vi "UI IO Page.vi"(8 "error in":errorcluster) -> (0 "error out":errorcluster)   [LabVIEW 2019, in "UIs.lvlib"]
uses:
  UIs.lvlib
  <vilib>/Utility/miscctls.llb/LVPointTypeDef.ctl
  LED/SubVI/ADC Channel.ctl
  Controller/Controller.lvlib
  IO/sbRIO9623/sbRIO9623.lvlib
  Selection Valve/IDEX/IDEX.lvlib
  Syringe Pump/NE-500/NE-500.lvlib
  LED/LED.lvlib
panel:
  out "Syringe Pump Status":string
  out "Force Sensor 2":u32
  out "Force Sensor 1":u32
  out "Air Pressure (V)":dbl format="%#_2g"
  out "Blood Sensor 2 (V)":dbl format="%#_2g"
  out "Blood Sensor 1 (V)":dbl format="%#_2g"
  out "BL1 (V)":dbl format="%#_2g"
  out "BL2 (V)":dbl format="%#_2g"
  in  "Back":bool
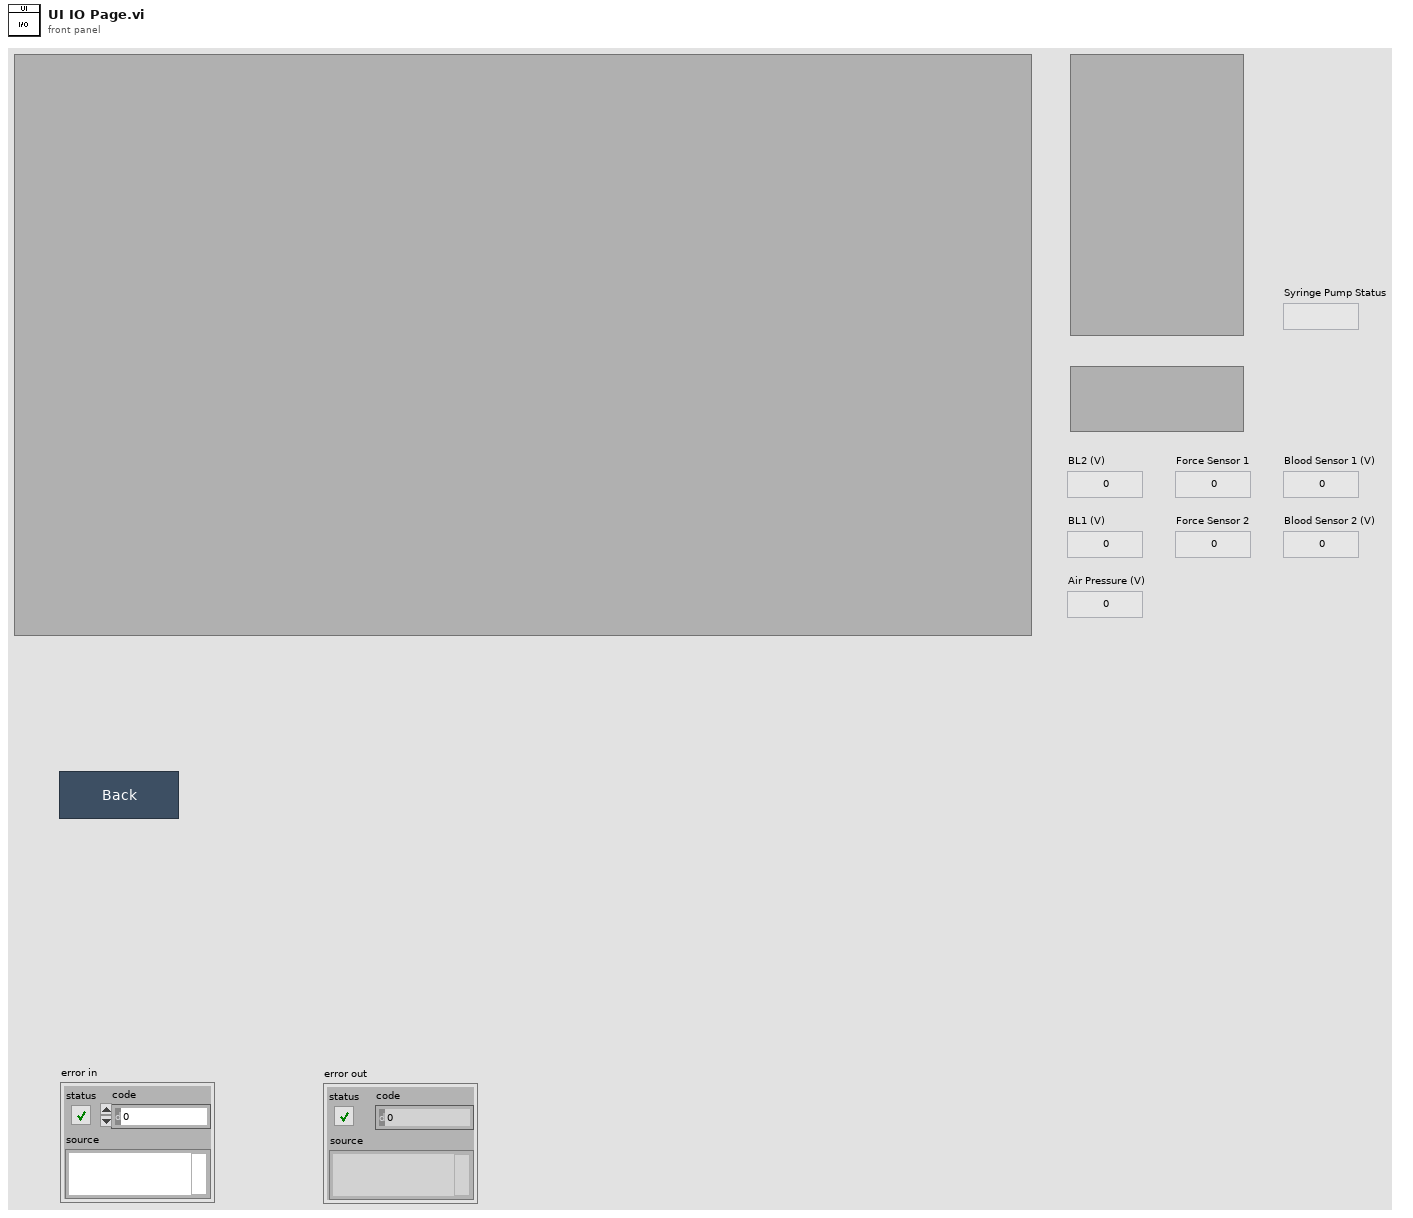
[diagram p1: front panel]
types:
  T1 = typedef "LVPointTypeDef.ctl" = cluster{"Horizontal":i16, "Vertical":i16}
  T2 = typedef "NE-500.lvlib/SEQ Data.ctl" = cluster{"Status":string, "Initialize Done?":bool, "VI Refnum":refnum<vi>}
  T3 = typedef "sbRIO9623.lvlib/SEQ Data.ctl" = cluster{"Lid Sensor 1":bool, "Lid Sensor 2":bool, "Laser Interlock":bool, "Buffer Tank":bool, "Wash Tank":bool, "Waste Tank":bool, "SiPM 1":fxp<+,20,5>, "SiPM 2":fxp<+,20,5>, "Initialize Success?":bool, "VI Refnum":refnum<vi>}
  T4 = typedef "IDEX.lvlib/SEQ Data.ctl" = cluster{"Position":string, "Initialize Done?":bool, "VI Refnum":refnum<vi>}
  T5 = typedef "LED.lvlib/ADC Channel.ctl" = enum16{"BL2 Regulator", "BL1 Regulator", "Blood Sensor 1", "Blood Sensor 2", "Air Pressure Sensor", "Force Sensor 1", "Force Snesor 2"}
  T6 = typedef "LED.lvlib/SEQ Data.ctl" = cluster{"Initialize Sucess?":bool, "BL2 Regulator":dbl, "BL1 Regulator":dbl, "Blood Sensor 1":dbl, "Blood Sensor 2":dbl, "Air Pressure Sensor":dbl, "Force Snesor 1":u32, "Force Snesor 2":u32, "VI Refnum":refnum<vi>}
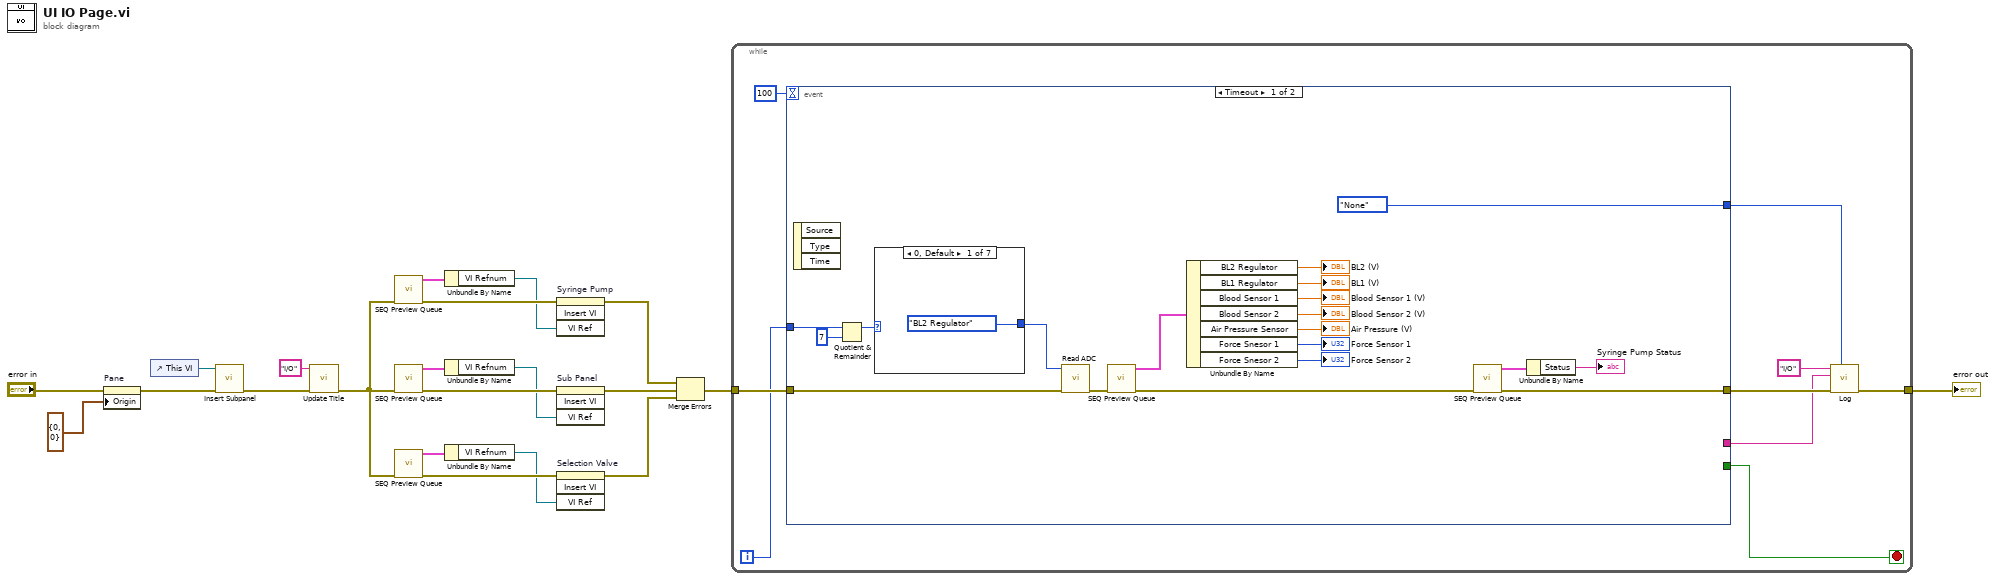
[diagram p0: block diagram]
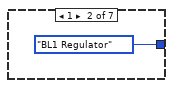
[diagram p2: hidden frame]
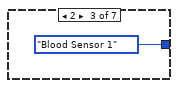
[diagram p3: hidden frame]
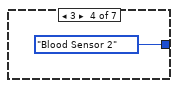
[diagram p4: hidden frame]
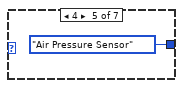
[diagram p5: hidden frame]
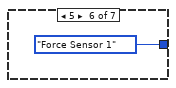
[diagram p6: hidden frame]
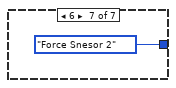
[diagram p7: hidden frame]
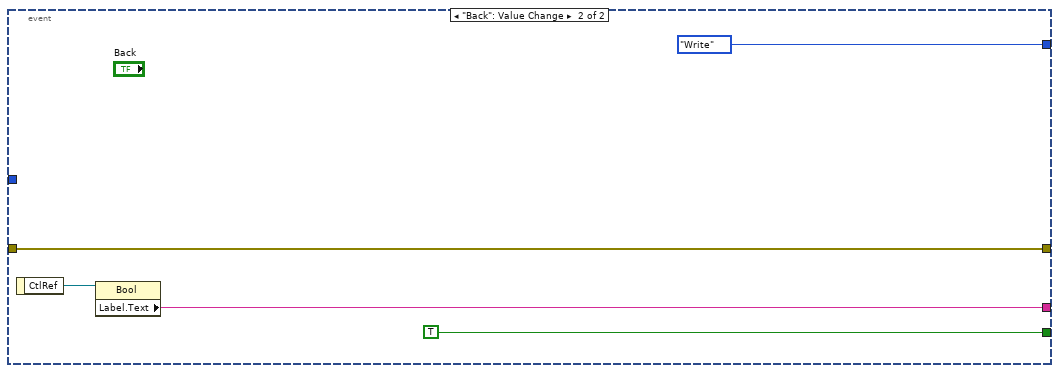
[diagram p8: hidden frame]
diagram:
  n1 = property on="Pane" class="Pane"(error in="error in", "Origin"=T1 {"Horizontal"=0, "Vertical"=0}) -> (error out=w15:errorcluster)  [unwired: 1 in, 1 out]
  n2 = control-ref of="This VI"() -> (w21:refnum<vi>)
  n3 = call "Insert Subpanel.vi"("Error In"=w15, "VI Refnum"=w21) -> ("Error Out"=w13:errorcluster)  [unwired: 9 in]
  n4 = call "Update Title.vi"("Error In"=w13, "Title"="I/O") -> ("Error Out"=w10:errorcluster)  [unwired: 9 in]
  n5 = call "SEQ Preview Queue.vi"("error in"=w10) -> ("error out"=w11:errorcluster, "SEQ Data"=w9:T2)  [unwired: 9 in]
  n6 = call "SEQ Preview Queue.vi"("error in"=w10) -> ("error out"=w19:errorcluster, "SEQ Data"=w20:T3)  [unwired: 9 in]
  n7 = call "SEQ Preview Queue.vi"("error in"=w10) -> ("error out"=w7:errorcluster, "SEQ Data"=w6:T4)  [unwired: 9 in]
  n8 = Unbundle By Name(w9) -> ("VI Refnum"=w8:refnum<vi>)
  n9 = Unbundle By Name(w20) -> ("VI Refnum"=w18:refnum<vi>)
  n10 = Unbundle By Name(w6) -> ("VI Refnum"=w5:refnum<vi>)
  n11 = invoke on="Syringe Pump" class="SubPnl" method="Insert VI"(error in=w11, "VI Ref"=w8) -> (error out=w4:errorcluster)  [unwired: 2 in, 3 out]
  n12 = invoke on="Sub Panel" class="SubPnl" method="Insert VI"(error in=w19, "VI Ref"=w18) -> (error out=w3:errorcluster)  [unwired: 2 in, 3 out]
  n13 = invoke on="Selection Valve" class="SubPnl" method="Insert VI"(error in=w7, "VI Ref"=w5) -> (error out=w2:errorcluster)  [unwired: 2 in, 3 out]
  n14 = Merge Errors(w4, w3, w2) -> (w1:errorcluster)
  n15 = while {
    tunnel: w1 -> [w30]
    tunnel: [w25] -> w17
    i -> [w28]
    stop <- w29 stop-if-true
    n16 = event shown="[0] Timeout" {
      selector: _ -> [_ _]
      dyn-events: _ -> [_ _]
      timeout: 100 -> [_ _]
      tunnel: w30 -> [w41 w61]
      tunnel: [w32 w61] -> w26
      tunnel: [_ TRUE] -> w29
      tunnel: w28 -> [w39 _]
      tunnel: [enum16{"None", "Write"}."None" ("Action") enum16{"None", "Write"}."Write" ("Action")] -> w24
      tunnel: [_ w58] -> w22
      event Timeout {
        n17 = event-data() -> ()  [unwired: 1 in, 3 out]
        n18 = Quotient & Remainder(x=w39, y=7) -> (x-y*floor(x/y)=w37:i32)  [unwired: 1 out]
        n19 = case shown="0, Default" w37 {
          tunnel: [ADC_Channel."BL2 Regulator" ("ADC Channel") ADC_Channel."BL1 Regulator" ("ADC Channel") ADC_Channel."Blood Sensor 1" ("ADC Channel") ADC_Channel."Blood Sensor 2" ("ADC Channel") ADC_Channel."Air Pressure Sensor" ("ADC Channel") ADC_Channel."Force Sensor 1" ("ADC Channel") ADC_Channel."Force Snesor 2" ("ADC Channel")] -> w36
          frame 0, Default {
          }
          frame 1 {
          }
          frame 2 {
          }
          frame 3 {
          }
          frame 4 {
          }
          frame 5 {
          }
          frame 6 {
          }
        }
        n20 = call "Read ADC.vi"("Error In"=w41, "ADC Channel"=w36) -> ("Error Out"=w40:errorcluster)  [unwired: 9 in]
        n21 = call "SEQ Preview Queue.vi"("error in"=w40) -> ("error out"=w33:errorcluster, "SEQ Data"=w42:T6)  [unwired: 9 in]
        n22 = Unbundle By Name(w42) -> ("BL2 Regulator"=→"BL2 (V)":dbl, "BL1 Regulator"=→"BL1 (V)":dbl, "Blood Sensor 1"=→"Blood Sensor 1 (V)":dbl, "Blood Sensor 2"=→"Blood Sensor 2 (V)":dbl, "Air Pressure Sensor"=→"Air Pressure (V)":dbl, "Force Snesor 1"=→"Force Sensor 1":u32, "Force Snesor 2"=→"Force Sensor 2":u32)
        n23 = call "SEQ Preview Queue.vi"("error in"=w33) -> ("error out"=w32:errorcluster, "SEQ Data"=w34:T2)  [unwired: 9 in]
        n24 = Unbundle By Name(w34) -> ("Status"=→"Syringe Pump Status":string)
      }
      event "Back": Value Change {
        n25 = event-data() -> ("CtlRef"=w59:refnum<vi>)  [unwired: 1 in]
        n26 = property class="Bool"(reference=w59) -> ("Label.Text"=w58:string)  [unwired: 1 in, 2 out]
      }
    }
    n27 = call "Log.vi"("Action"=w24, "error in"=w26, "State"=w22, "Page Name"="I/O") -> ("error out"=w25:errorcluster)  [unwired: 7 in]
  }
  "error out" <- w17
